vi "gfitsio-open-create-replace-image.vi"(4 "image data type":T1 items=["<invalid type>"=0, "BYTE_IMG  (U8)"=8, "SHORT_IMG  (I16)"=16, "USHORT_IMG  (U16)"=20, "LONG_IMG  (I32)"=32, "ULONG_IMG  (U32)"=40, "FLOAT_IMG  (SGL)"=-32, "DOUBLE_IMG  (DBL)"=-64], 5 "prompt (\"Select an HDU\")":string="Select an HDU", 6 "advisory dialog? (display:T)":bool=TRUE, 7 "hdu name (dialog if empty)":string, 8 "error in (no error)":errorcluster, 9 "function (create or replace)":T3(ring)=enum."create or replace", 10 "naxes":i32[](array[numeric]), 11 "gfits refnum":T2) -> (0 "error out":errorcluster, 2 "hdu name out":string, 3 "dup gfits refnum":T2)   [LabVIEW 2019, in "gfitsio.lvlib"]
doc: "Opens an existing FITS image HDU, creates a new FITS image HDU, or replaces an existing FITS image HDU, programmatically or interactively using a dialog box. You can optionally specify a dialog prompt."
uses:
  gfitsio.lvlib
  gfitsio-refnum.ctl
  cfitsio-bitpix.ctl
  cfitsio-hdutypes.ctl
  gfitsio-error-codes.ctl
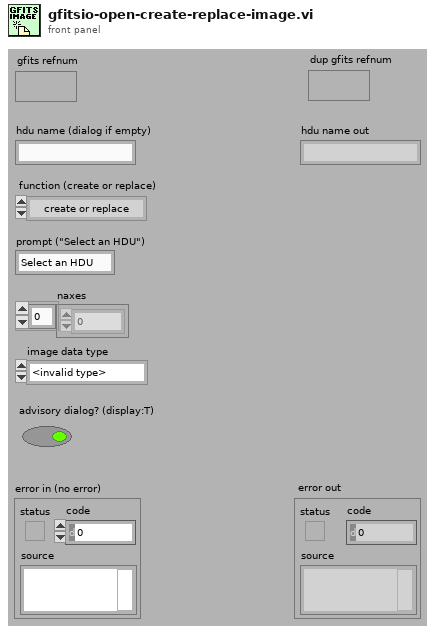
[diagram p1: front panel]
types:
  T1 = typedef "gfitsio.lvlib/cfitsio-bitpix.ctl" = i32
  T2 = typedef "gfitsio.lvlib/gfitsio-refnum.ctl" = refnum<k1>
  T3 = enum16{"open", "open or create", "create", "create or replace"}
  T4 = typedef "gfitsio.lvlib/cfitsio-hdutypes.ctl" = i32
  T5 = typedef "gfitsio.lvlib/gfitsio-error-codes.ctl" = i32
  T6 = enum16{"Error", "Ok", "Cancel", "Abort", "Retry", "Ignore", "Yes", "No", "Close", "Help", "Disabled"}
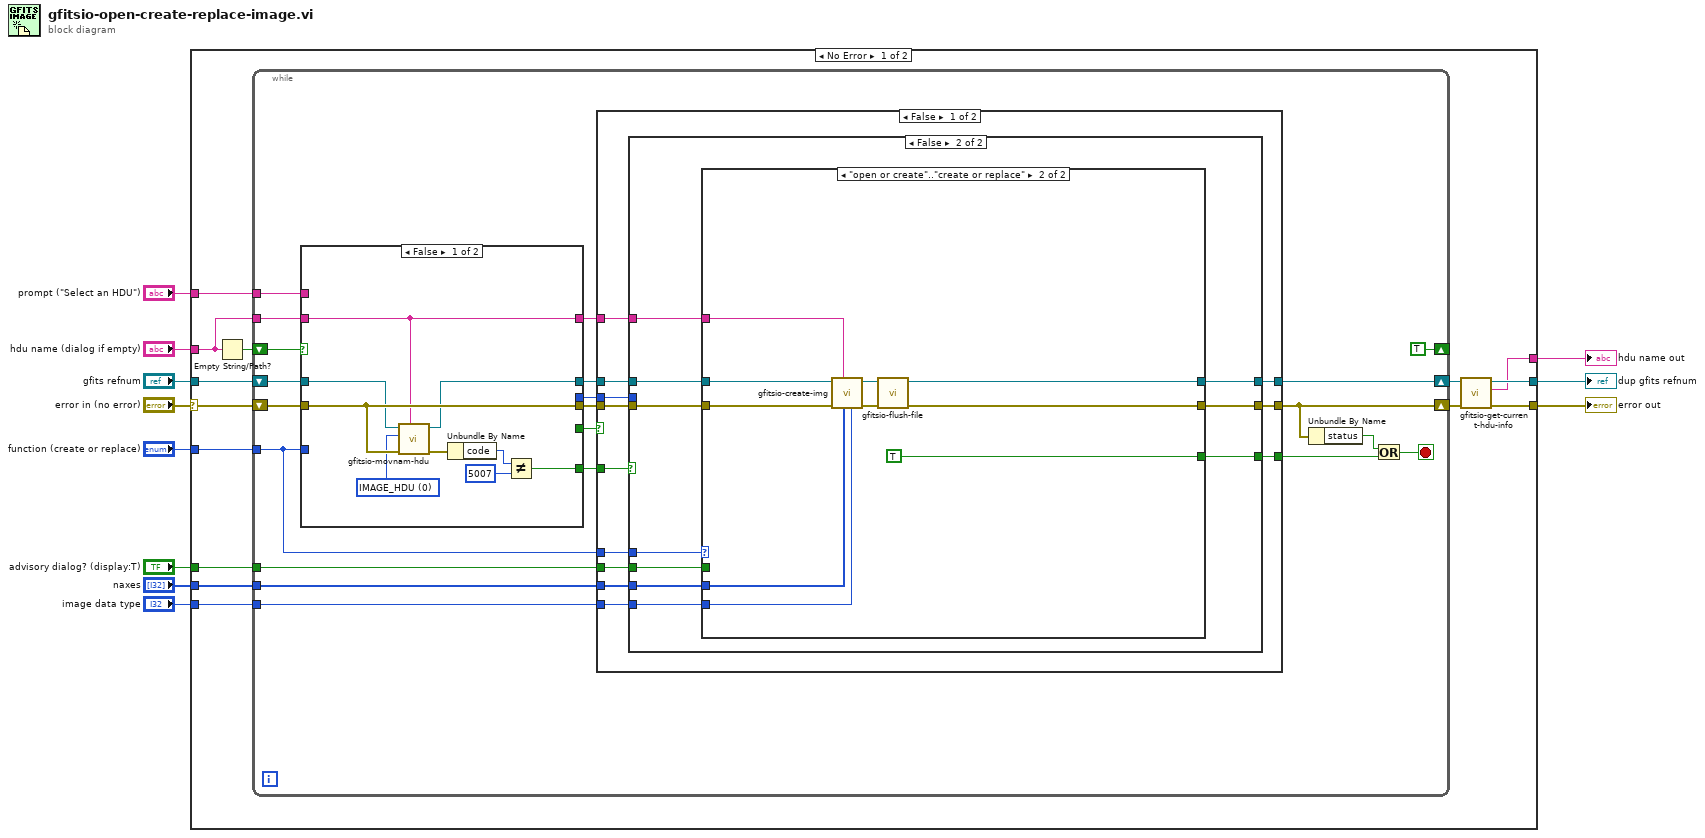
[diagram p0: block diagram]
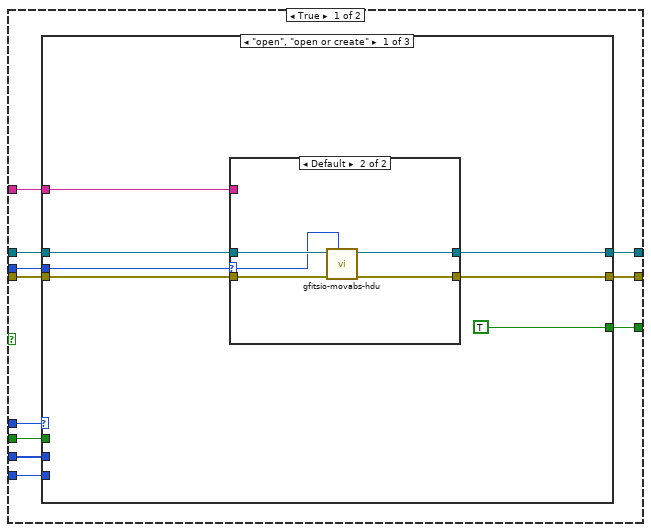
[diagram p2: hidden frame]
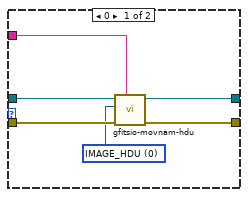
[diagram p3: hidden frame]
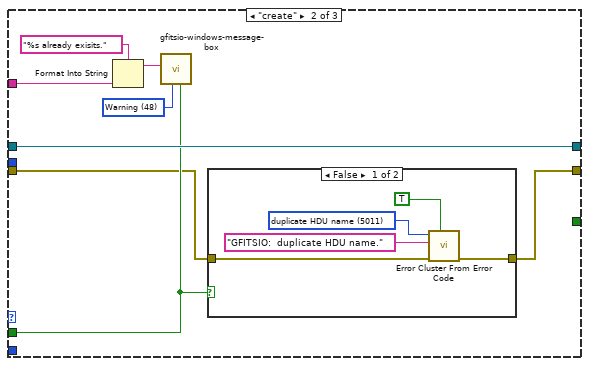
[diagram p4: hidden frame]
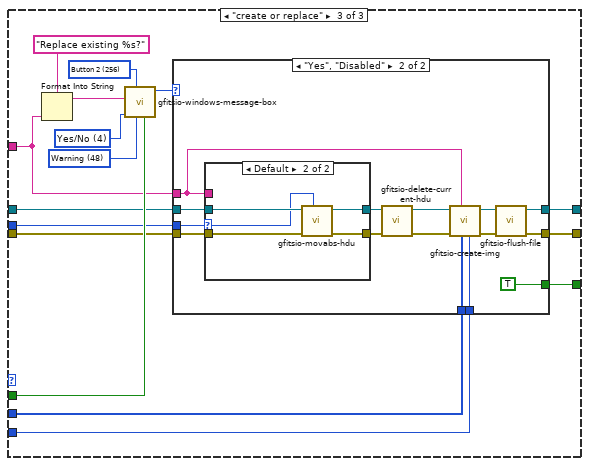
[diagram p6: hidden frame]
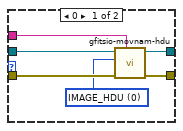
[diagram p8: hidden frame]
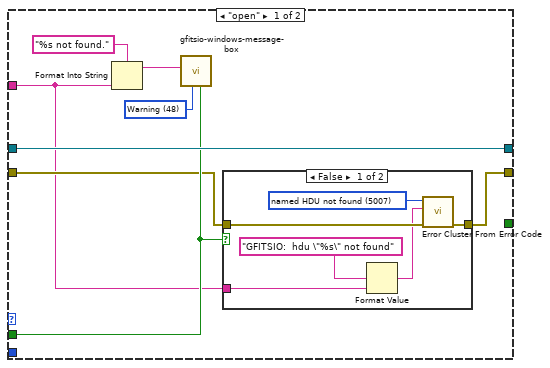
[diagram p9: hidden frame]
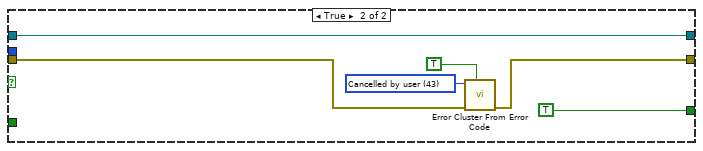
[diagram p11: hidden frame]
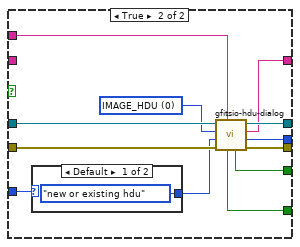
[diagram p12: hidden frame]
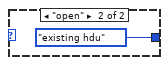
[diagram p13: hidden frame]
diagram:
  n1 = case shown="No Error" "error in (no error)" {
    selector: "error in (no error)" -> [w12 w210]
    tunnel: "advisory dialog? (display:T)" -> [w24 _]
    tunnel: "function (create or replace)" -> [w23 _]
    tunnel: "prompt (\"Select an HDU\")" -> [w22 _]
    tunnel: "hdu name (dialog if empty)" -> [w21 _]
    tunnel: "gfits refnum" -> [w20 w211]
    tunnel: [w17 w210] -> w6
    tunnel: [w16 w211] -> w5
    tunnel: [w15 _] -> w4
    tunnel: "naxes" -> [w14 _]
    tunnel: "image data type" -> [w13 _]
    frame No Error {
      n2 = Empty String/Path?(string/path=w21) -> (empty?=w25:bool)
      n3 = while {
        tunnel: w23 -> [w30]
        shift-right: [w39] -> w18
        shift-left: w12 -> [w46]
        shift-right: [w42] -> w19
        shift-left: w20 -> [w45]
        tunnel: w21 -> [w34]
        tunnel: w22 -> [w31]
        tunnel: w24 -> [w29]
        tunnel: w14 -> [w28]
        tunnel: w13 -> [w27]
        shift-right: [TRUE] -> _
        shift-left: w25 -> [w44]
        stop <- w36 stop-if-true
        n4 = case shown="False" w44 {
          tunnel: [w195 w207] -> w41
          tunnel: [w193 w206] -> w43
          tunnel: w46 -> [w195 w205]
          tunnel: w45 -> [w194 w204]
          tunnel: w30 -> [_ w203]
          tunnel: [_ w202] -> w40
          tunnel: [w189 w201] -> w35
          tunnel: w34 -> [w188 _]
          tunnel: [w188 w200] -> w33
          tunnel: [_ w199] -> w32
          tunnel: w31 -> [_ w198]
          frame False {
            w187 = T4 0 items=["ANY_HDU"=-1, "IMAGE_HDU"=0, "ASCII_TBL"=1, "BINARY_TBL"=2] ("hdu type (ANY)")
            n5 = call "gfitsio-movnam-hdu.vi"("extname"=w188, "error in (no error)"=w195, "hdutype (ANY_HDU)"=w187, "gfits refnum"=w194) -> ("error out"=w192:errorcluster, "dup gfits refnum"=w193:T2)  [unwired: 2 in, 4 out]
            n6 = Unbundle By Name(w192) -> ("code"=w191:i32)
            n7 = Not Equal?(x=w191, y=5007) -> (x != y?=w189:bool)
          }
          frame True {
            w196 = T4 0 items=["ANY_HDU"=-1, "IMAGE_HDU"=0, "ASCII_TBL"=1, "BINARY_TBL"=2] ("hdu type (ANY)")
            n8 = case shown="Default" w203 {
              tunnel: [enum32{"existing hdu", "new or existing hdu"}."new or existing hdu" ("select mode (new or existing)") enum32{"existing hdu", "new or existing hdu"}."existing hdu" ("select mode (new or existing)")] -> w197
              frame Default {
              }
              frame "open" {
              }
            }
            n9 = call "gfitsio-hdu-dialog.vi"("prompt (\"Select an HDU\")"=w198, "error in (no error)"=w205, "select mode (new or existing)"=w197, "hdu type (ANY_HDU)"=w196, "gfits refnum"=w204) -> ("error out"=w207:errorcluster, "hdu number (0 if cancelled)"=w199:i32, "hdu name (\"\" if cancelled)"=w200:string, "dup gfits refnum"=w206:T2, "cancelled"=w202:bool, "exists"=w201:bool)  [unwired: 1 out]
          }
        }
        n10 = case shown="False" w40 {
          tunnel: w43 -> [w58 w186]
          tunnel: [w55 w186] -> w42
          tunnel: w41 -> [w57 w182]
          tunnel: [w56 w181] -> w39
          tunnel: [w49 TRUE] -> w37
          tunnel: w35 -> [w54 _]
          tunnel: w33 -> [w52 _]
          tunnel: w32 -> [w51 _]
          tunnel: w30 -> [w53 _]
          tunnel: w29 -> [w50 _]
          tunnel: w28 -> [w48 _]
          tunnel: w27 -> [w47 _]
          frame False {
            n11 = case shown="False" w54 {
              tunnel: w58 -> [w68 w154]
              tunnel: w57 -> [w65 w153]
              tunnel: [w66 w152] -> w56
              tunnel: [w67 w151] -> w55
              tunnel: w53 -> [w69 w155]
              tunnel: w52 -> [w64 w149]
              tunnel: w51 -> [w63 _]
              tunnel: w50 -> [w62 w150]
              tunnel: [w61 w148] -> w49
              tunnel: w48 -> [w60 w147]
              tunnel: w47 -> [w59 w146]
              frame True {
                n12 = case shown="\"open\", \"open or create\"" w69 {
                  tunnel: w68 -> [w75 w95 w111]
                  tunnel: [w73 w95 w110] -> w67
                  tunnel: [w74 w88 w108] -> w66
                  tunnel: w65 -> [w76 w89 w109]
                  tunnel: w64 -> [w72 w91 w105]
                  tunnel: w63 -> [w71 _ w104]
                  tunnel: w62 -> [_ w90 w112]
                  tunnel: [TRUE _ w106] -> w61
                  tunnel: w60 -> [_ _ w103]
                  tunnel: w59 -> [_ _ w102]
                  frame "open", "open or create" {
                    n13 = case shown="Default" w71 {
                      selector: w71 -> [_ w83]
                      tunnel: w76 -> [w82 w86]
                      tunnel: w75 -> [w81 w87]
                      tunnel: [w80 w85] -> w74
                      tunnel: [w79 w84] -> w73
                      tunnel: w72 -> [w78 _]
                      frame 0 {
                        w77 = T4 0 items=["ANY_HDU"=-1, "IMAGE_HDU"=0, "ASCII_TBL"=1, "BINARY_TBL"=2] ("hdu type (ANY)")
                        n14 = call "gfitsio-movnam-hdu.vi"("extname"=w78, "error in (no error)"=w82, "hdutype (ANY_HDU)"=w77, "gfits refnum"=w81) -> ("error out"=w80:errorcluster, "dup gfits refnum"=w79:T2)  [unwired: 2 in, 4 out]
                      }
                      frame Default {
                        n15 = call "gfitsio-movabs-hdu.vi"("hdunum"=w83, "error in (no error)"=w86, "gfits refnum"=w87) -> ("error out"=w85:errorcluster, "dup gfits refnum"=w84:T2)  [unwired: 1 in, 6 out]
                      }
                    }
                  }
                  frame "create" {
                    w92 = u32 48 items=["None"=0, "Warning"=48, "Confirmation"=64, "Question"=32, "Error"=16, "User Icon"=128] ("Icon (None)")
                    n16 = Format Into String(format string="%s already exisits.", w91) -> (resulting string=w93:string)  [unwired: 2 in, 1 out]
                    n17 = call "gfitsio-windows-message-box.vi"("enable dialog?"=w90, "Icon (None)"=w92, "Text"=w93) -> ()  [unwired: 4 in, 5 out]
                    n18 = case shown="False" w90 {
                      tunnel: w89 -> [w100 w101]
                      tunnel: [w99 w101] -> w88
                      frame False {
                        w96 = T5 5011 items=["no error"=0, "dimensionality conflict"=5001, "fpixel out of image bounds"=5002, "lpixel out of image bounds"=5003, "increment size larger than image"=5004, "increment must be greater than zero"=5005, "fpixel must specify lower left corner"=5006, "named HDU not found"=5007, "specified row is past the end of the table"=5008, "wrong number of elements for column"=5009, "column is not scalar"=5010, "duplicate HDU name"=5011, "invalid table type"=5012] ("Ring")
                        n19 = call <vilib>:"Error Cluster From Error Code.vi"("show call chain? (False)"=TRUE, "error in (no error)"=w100, "error message (\"\")"="GFITSIO:  duplicate HDU name." ("error message (\"\")"), "error code (0)"=w96) -> ("error out"=w99:errorcluster)  [unwired: 5 out]
                      }
                      frame True {
                      }
                    }
                  }
                  frame "create or replace" {
                    w114 = u32 256 items=["Button 1"=0, "Button 2"=256, "Button 3"=512, "Button 4"=1024] ("Default (Button 1)")
                    w115 = u32 4 items=["Abort/Retry/Ignore"=2, "OK"=0, "OK/Cancel"=1, "Retry/Cancel"=5, "Yes/No"=4, "Yes/No/Cancel"=3] ("Buttons (OK)")
                    w116 = u32 48 items=["None"=0, "Warning"=48, "Confirmation"=64, "Question"=32, "Error"=16, "User Icon"=128] ("Icon (None)")
                    n20 = Format Into String(format string="Replace existing %s?", w105) -> (resulting string=w113:string)  [unwired: 2 in, 1 out]
                    n21 = call "gfitsio-windows-message-box.vi"("enable dialog?"=w112, "Icon (None)"=w116, "Default (Button 1)"=w114, "Buttons (OK)"=w115, "Text"=w113) -> ("Button Selected"=w107:T6)  [unwired: 3 in, 3 out]
                    n22 = case shown="\"Yes\", \"Disabled\"" w107 {
                      tunnel: w111 -> [w119 w133]
                      tunnel: [w119 w124] -> w110
                      tunnel: w109 -> [w118 w132]
                      tunnel: [w118 w123] -> w108
                      tunnel: [_ TRUE] -> w106
                      tunnel: w105 -> [_ w122]
                      tunnel: w104 -> [_ w131]
                      tunnel: w103 -> [_ w121]
                      tunnel: w102 -> [_ w120]
                      frame "No", Default {
                      }
                      frame "Yes", "Disabled" {
                        n23 = case shown="Default" w131 {
                          selector: w131 -> [_ w141]
                          tunnel: w132 -> [w140 w144]
                          tunnel: w133 -> [w139 w145]
                          tunnel: [w138 w143] -> w130
                          tunnel: [w137 w142] -> w129
                          tunnel: w122 -> [w136 _]
                          frame 0 {
                            w135 = T4 0 items=["ANY_HDU"=-1, "IMAGE_HDU"=0, "ASCII_TBL"=1, "BINARY_TBL"=2] ("hdu type (ANY)")
                            n24 = call "gfitsio-movnam-hdu.vi"("extname"=w136, "error in (no error)"=w140, "hdutype (ANY_HDU)"=w135, "gfits refnum"=w139) -> ("error out"=w138:errorcluster, "dup gfits refnum"=w137:T2)  [unwired: 2 in, 4 out]
                          }
                          frame Default {
                            n25 = call "gfitsio-movabs-hdu.vi"("hdunum"=w141, "error in (no error)"=w144, "gfits refnum"=w145) -> ("error out"=w143:errorcluster, "dup gfits refnum"=w142:T2)  [unwired: 1 in, 6 out]
                          }
                        }
                        n26 = call "gfitsio-delete-current-hdu.vi"("error in (no error)"=w130, "gfits refnum"=w129) -> ("error out"=w127:errorcluster, "dup gfits refnum"=w128:T2)  [unwired: 8 out]
                        n27 = call "gfitsio-create-img.vi"("image data type"=w120, "naxes"=w121, "extname"=w122, "error in (no error)"=w127, "gfits refnum"=w128) -> ("error out"=w126:errorcluster, "dup gfits refnum"=w125:T2)  [unwired: 2 in, 3 out]
                        n28 = call "gfitsio-flush-file.vi"("error in (no error)"=w126, "gfits refnum"=w125) -> ("error out"=w123:errorcluster, "dup gfits refnum"=w124:T2)  [unwired: 8 out]
                      }
                    }
                  }
                }
              }
              frame False {
                n29 = case shown="\"open or create\"..\"create or replace\"" w155 {
                  tunnel: w154 -> [w163 w179]
                  tunnel: w153 -> [w158 w180]
                  tunnel: [w157 w175] -> w152
                  tunnel: [w163 w174] -> w151
                  tunnel: w150 -> [w159 _]
                  tunnel: w149 -> [w156 w173]
                  tunnel: [_ TRUE] -> w148
                  tunnel: w147 -> [_ w172]
                  tunnel: w146 -> [_ w171]
                  frame "open" {
                    w160 = u32 48 items=["None"=0, "Warning"=48, "Confirmation"=64, "Question"=32, "Error"=16, "User Icon"=128] ("Icon (None)")
                    n30 = Format Into String(format string="%s not found.", w156) -> (resulting string=w161:string)  [unwired: 2 in, 1 out]
                    n31 = call "gfitsio-windows-message-box.vi"("enable dialog?"=w159, "Icon (None)"=w160, "Text"=w161) -> ()  [unwired: 4 in, 5 out]
                    n32 = case shown="False" w159 {
                      tunnel: w158 -> [w169 w170]
                      tunnel: [w168 w170] -> w157
                      tunnel: w156 -> [w166 _]
                      frame False {
                        w164 = T5 5007 items=["no error"=0, "dimensionality conflict"=5001, "fpixel out of image bounds"=5002, "lpixel out of image bounds"=5003, "increment size larger than image"=5004, "increment must be greater than zero"=5005, "fpixel must specify lower left corner"=5006, "named HDU not found"=5007, "specified row is past the end of the table"=5008, "wrong number of elements for column"=5009, "column is not scalar"=5010, "duplicate HDU name"=5011, "invalid table type"=5012] ("Ring")
                        n33 = Format Value(format string="GFITSIO:  hdu \"%s\" not found", value (0)=w166) -> (output string=w165:string)  [unwired: 1 out]
                        n34 = call <vilib>:"Error Cluster From Error Code.vi"("error in (no error)"=w169, "error message (\"\")"=w165, "error code (0)"=w164) -> ("error out"=w168:errorcluster)  [unwired: 1 in, 5 out]
                      }
                      frame True {
                      }
                    }
                  }
                  frame "open or create".."create or replace" {
                    n35 = call "gfitsio-create-img.vi"("image data type"=w171, "naxes"=w172, "extname"=w173, "error in (no error)"=w180, "gfits refnum"=w179) -> ("error out"=w177:errorcluster, "dup gfits refnum"=w176:T2)  [unwired: 2 in, 3 out]
                    n36 = call "gfitsio-flush-file.vi"("error in (no error)"=w177, "gfits refnum"=w176) -> ("error out"=w175:errorcluster, "dup gfits refnum"=w174:T2)  [unwired: 8 out]
                  }
                }
              }
            }
          }
          frame True {
            w184 = 43 items=["No error", "Argument error", "Memory is full", "Out of zone", "End of file", "File already open", "Generic file I/O error", "File not found", "File permission error", "Disk is full", "Duplicate path", "Too many files open", "System feature not enabled", "Resource file not found", "Cannot add resource", "Resource not found", "Image not found", "Image memory error", "Pen does not exist", "Config type invalid", "Config token not found", "Config parse error", "Config memory error", "Bad external code format", "Bad external code offset", "External code not present", "Null window", "Destroy window error", "Null menu", "Print aborted", "Bad print record", "Print driver error", "Windows error during printing", "Memory error during printing", "Print dialog error", "Generic print error", "Invalid device refnum", "Device not found", "Device parameter error", "Device unit error", "Cannot open device", "Device call aborted", "Generic error", "Cancelled by user", "Object ID too low", "Object ID too high", "Object not in heap", "Unknown heap", "Unknown object (invalid DefProc)", "Unknown object (DefProc not in table)", "Message out of range", "Invalid (null) method", "Unknown message", "Manager call not supported", "Bad address", "Network operation in progress", "Network operation timed out", "Connection is busy", "Network attribute not supported", "Network error", "Address in use", "System out of memory", "Connection aborted", "Connection refused", "Not connected", "Already connected", "Connection closed", "Initialization error (interapplication manager)", "Bad occurrence", "Wait on unbound occurrence handler", "Occurrence queue overflow", "Datalog type conflict", "Unused", "Unrecognized type (interapplication manager)", "Memory corrupt", "Failed to make temporary DLL", "Old CIN version", "Drag socket not found", "Failed to load drop-object", "Failed to register OLE object", "Failed to release OLE object", "Format specifier type mismatch", "Unknown format specifier", "Too few format specifiers", "Too many format specifiers", "Scan failed", "Newer CIN version", "Error converting to variant", "Runtime menu error", "Password tampered", "Variant attribute not found", "Incompatible variant data type", "Event data is not available", "Event Store is not present", "Occurrence is not found", "Event Queue is not created", "Event info is not available in the type library", "Refnum passed is NULL", "Error retrieving Class GUID", "Error retrieving CoClass GUID", "Error retrieving TypeLib GUID.", "Bad built application magic bytes.", "Specific driver is different from the specific driver associated with the Logical Name.", "There is no session opened to the class driver.", "Max Error", "MAX - Error with config objects", "MAX - Error loading configuration", "MAX - Group not supported", "Singlecast connections can not send to multicast addresses.", "Multicast connections can not send to singlecast addresses.", "Specified IP address not in multicast address range.", "Attempt to write to read-only multicast connection.", "Attempt to read from write-only multicast connection.", "The buffer used to receive a datagram was smaller than the datagram itself"]
            n37 = call <vilib>:"Error Cluster From Error Code.vi"("show call chain? (False)"=TRUE, "error in (no error)"=w182, "error code (0)"=w184) -> ("error out"=w181:errorcluster)  [unwired: 6 out]
          }
        }
        n38 = Unbundle By Name(w39) -> ("status"=w38:bool)
        n39 = Or(x=w38, y=w37) -> (x .or. y?=w36:bool)
      }
      n40 = call "gfitsio-get-current-hdu-info.vi"("error in (no error)"=w18, "gfits refnum"=w19) -> ("error out"=w17:errorcluster, "hdu name"=w15:string, "dup gfits refnum"=w16:T2)  [unwired: 1 in, 6 out]
    }
    frame Error {
    }
  }
  "error out" <- w6
  "dup gfits refnum" <- w5
  "hdu name out" <- w4
